vi "Waveform_Intensity_Graph.vi"(6 "error in":errorcluster) -> (0 "Intensity Graph Ch1":dbl[][](graph), 3 "Intensity Graph Ch2":dbl[][](graph))   [LabVIEW 2019]
uses:
  <vilib>/Utility/error.llb/DialogType.ctl
  ESA_Data_Analysis_Global_VIs.vi
  SiPM_Tests_Global_Var.vi
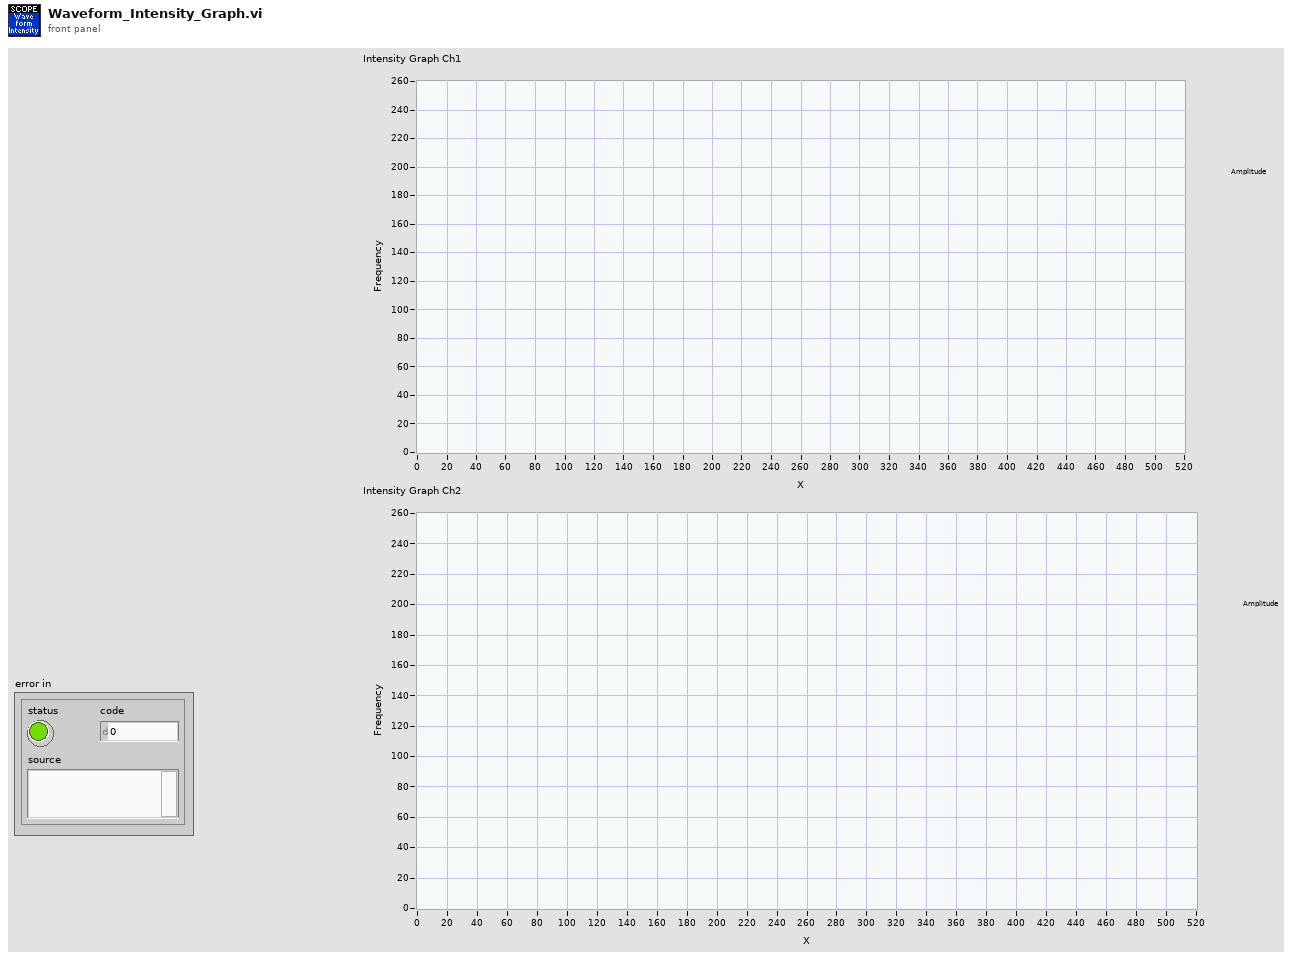
[diagram p1: front panel]
types:
  T1 = typedef "DialogType.ctl" = u16
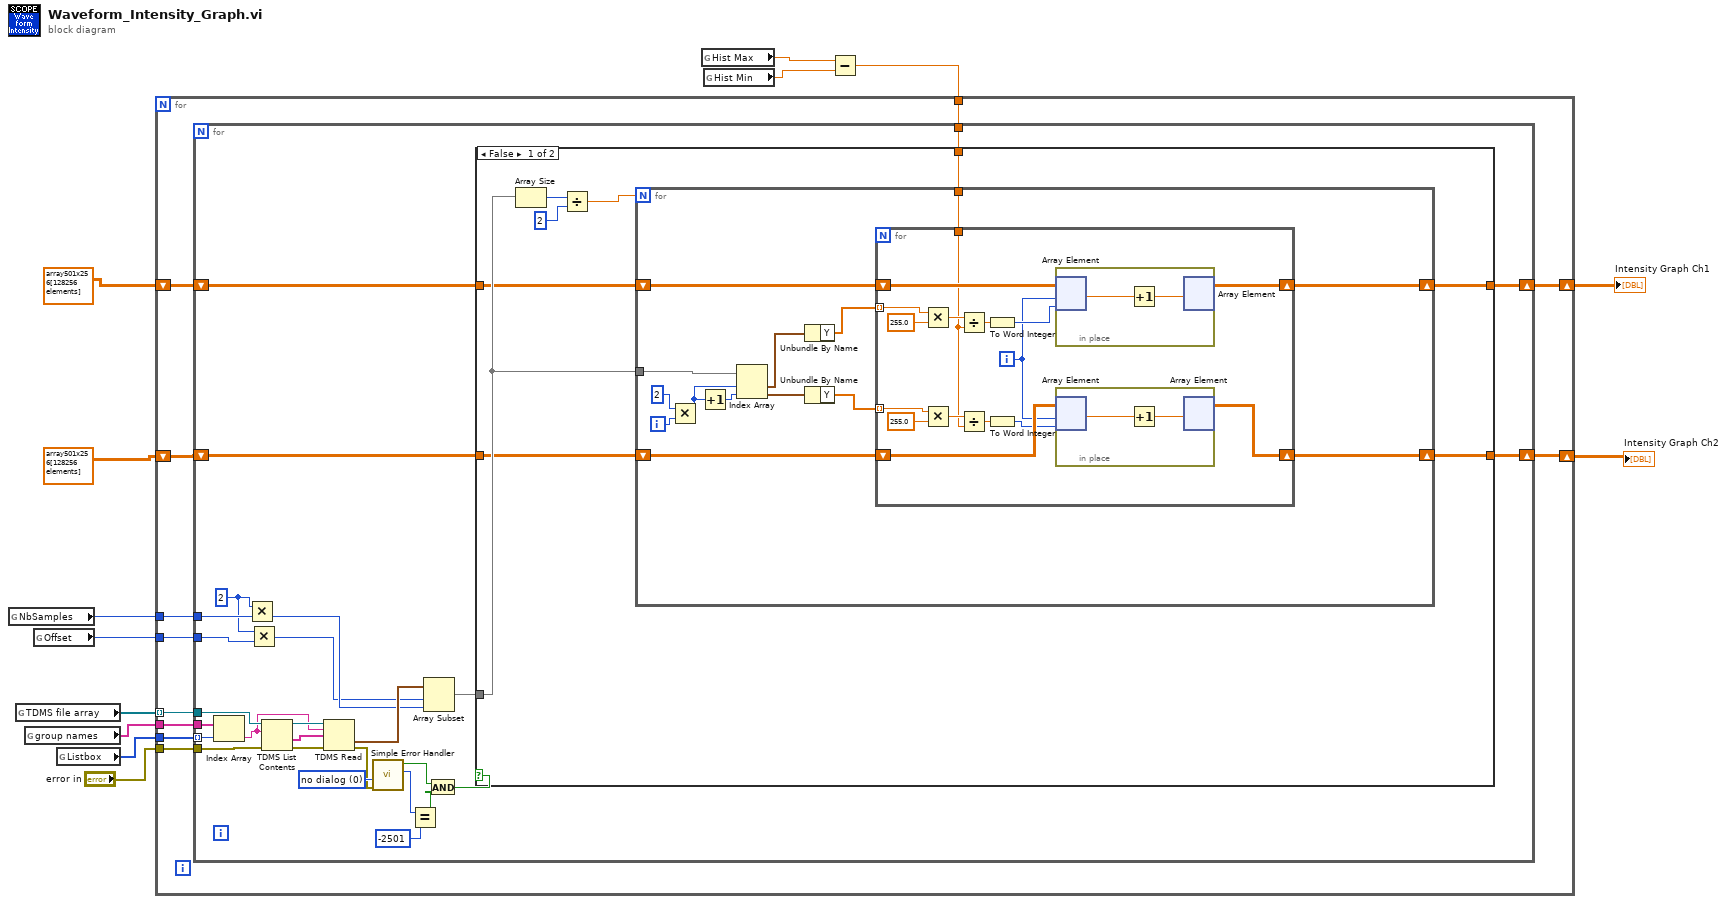
[diagram p0: block diagram]
diagram:
  n1 = global read "SiPM_Tests_Global_Var.vi" "NbSamples"() -> (w8:i64)
  n2 = global read "SiPM_Tests_Global_Var.vi" "TDMS file array"() -> (w10:refnum<k34>[])
  n3 = global read "ESA_Data_Analysis_Global_VIs.vi" "group names"() -> (w13:string[])
  n4 = global read "SiPM_Tests_Global_Var.vi" "Offset"() -> (w9:i64)
  n5 = global read "ESA_Data_Analysis_Global_VIs.vi" "Listbox"() -> (w12:i32[])
  n6 = global read "SiPM_Tests_Global_Var.vi" "Hist Max"() -> (w3:dbl)
  n7 = global read "SiPM_Tests_Global_Var.vi" "Hist Min"() -> (w2:dbl)
  n8 = Subtract(x=w3, y=w2) -> (x-y=w1:dbl)
  n9 = for {
    tunnel: w10 -> [w24] mode=indexing
    tunnel: w13 -> [w23]
    tunnel: w12 -> [w22]
    tunnel: "error in" -> [w21]
    tunnel: w9 -> [w20]
    tunnel: w8 -> [w19]
    shift-right: [w17] -> w5
    shift-left: dbl[][] array501x256[128256 elements] -> [w18]
    shift-right: [w15] -> w4
    shift-left: dbl[][] array501x256[128256 elements] -> [w16]
    tunnel: w1 -> [w14]
    n10 = for {
      tunnel: w24 -> [w51]
      tunnel: w23 -> [w50]
      tunnel: w22 -> [w49] mode=indexing
      tunnel: w21 -> [w48]
      tunnel: w20 -> [w35]
      tunnel: w19 -> [w34]
      shift-right: [w28] -> w17
      shift-left: w18 -> [w29]
      shift-right: [w26] -> w15
      shift-left: w16 -> [w27]
      tunnel: w14 -> [w25]
      w30 = i64 2 ("x")
      w45 = T1 0 items=["no dialog", "OK message", "continue or stop message", "OK message + warnings", "continue/stop + warnings"] ("type of dialog (OK msg:1)")
      n11 = Index Array(array=w50, index=w49) -> (element=w46:string)
      n12 = Multiply(x=w30, y=w34) -> (x*y=w32:i64)
      n13 = Multiply(x=w30, y=w35) -> (x*y=w31:i64)
      n14 = TDMS List Contents(4:w48, 6:w46, 7:w51) -> (0:w42:errorcluster, 1:w43:string[], 3:w47:refnum<k34>)  [unwired: 1 out]
      n15 = TDMS Read(0:w47, 5:w46, 7:w43, 11:w42) -> (10:w36:waveform(dbl)[], 15:w44:errorcluster)  [unwired: 4 in, 4 out]
      n16 = call <vilib>:"Simple Error Handler.vi"("type of dialog (OK msg:1)"=w45, "error in (no error)"=w44) -> ("error?"=w40:bool, "code out"=w39:i32)  [unwired: 3 in, 3 out]
      n17 = Equal?(x=w39, y=-2501) -> (x = y?=w37:bool)
      n18 = Array Subset(array=w36, index=w31, length=w32) -> (w33:waveform(dbl)[])
      n19 = And(x=w40, y=w37) -> (x .and. y?=w41:bool)
      n20 = case shown="False" w41 {
        tunnel: w33 -> [w57 _]
        tunnel: w29 -> [w56 w96]
        tunnel: [w55 w96] -> w28
        tunnel: w27 -> [w54 w95]
        tunnel: [w53 w95] -> w26
        tunnel: w25 -> [w52 _]
        frame False {
          n21 = Array Size(array=w57) -> (size(s)=w60:i32)
          n22 = Divide(x=w60, y=2) -> (x/y=w58:dbl)
          n23 = for {
            N: w58 -> [_]
            tunnel: w57 -> [w73]
            shift-right: [w66] -> w55
            shift-left: w56 -> [w67]
            shift-right: [w62] -> w53
            shift-left: w54 -> [w63]
            tunnel: w52 -> [w61]
            i -> [w70]
            n24 = Multiply(x=2, y=w70) -> (x*y=w71:i32)
            n25 = Increment(x=w71) -> (x+1=w74:i32)
            n26 = Index Array(array=w73, index #1=w71, index #2=w74) -> (element #1=w69:waveform(dbl), element #2=w65:waveform(dbl))
            n27 = Unbundle By Name(w69) -> ("Y"=w68:dbl[])
            n28 = Unbundle By Name(w65) -> ("Y"=w64:dbl[])
            n29 = for {
              tunnel: w68 -> [w86] mode=indexing
              shift-right: [w89] -> w66
              shift-left: w67 -> [w90]
              tunnel: w64 -> [w76] mode=indexing
              shift-right: [w87] -> w62
              shift-left: w63 -> [w88]
              tunnel: w61 -> [w75]
              i -> [w78]
              n30 = Multiply(x=w86, y=255.0) -> (x*y=w84:dbl)
              n31 = Multiply(x=w76, y=255.0) -> (x*y=w80:dbl)
              n32 = Divide(x=w84, y=w75) -> (x/y=w83:dbl)
              n33 = Divide(x=w80, y=w75) -> (x/y=w81:dbl)
              n34 = To Word Integer(number=w83) -> (16bit integer=w82:i16)
              n35 = To Word Integer(number=w81) -> (16bit integer=w77:i16)
              n36 = in-place {
                n37 = in-place-array #1(w90, w78, w82) -> (w94:dbl)
                n38 = Increment(x=w94) -> (x+1=w93:dbl)
                n39 = in-place-array #1(w93) -> (w89:dbl[][])  [unwired: 2 out]
              }
              n40 = in-place {
                n41 = in-place-array #2(w88, w78, w77) -> (w92:dbl)
                n42 = Increment(x=w92) -> (x+1=w91:dbl)
                n43 = in-place-array #2(w91) -> (w87:dbl[][])  [unwired: 2 out]
              }
            }
          }
        }
        frame True {
        }
      }
    }
  }
  "Intensity Graph Ch1" <- w5
  "Intensity Graph Ch2" <- w4
